vi "Write Output waveform.vi"(8 "error in (no error)":errorcluster, 10 "Output waveform":i16[](array[numeric]), 11 "RP I-V Driver in":refnum<class "RP I-V Driver.lvclass">) -> (0 "error out":errorcluster, 3 "RP I-V Driver out":refnum<class "RP I-V Driver.lvclass">)   [LabVIEW 2016, in "RP I-V Driver.lvclass"]
uses:
  RP I-V Driver.lvclass
  RP I-V Driver.lvclass/RP I-V Driver.ctl
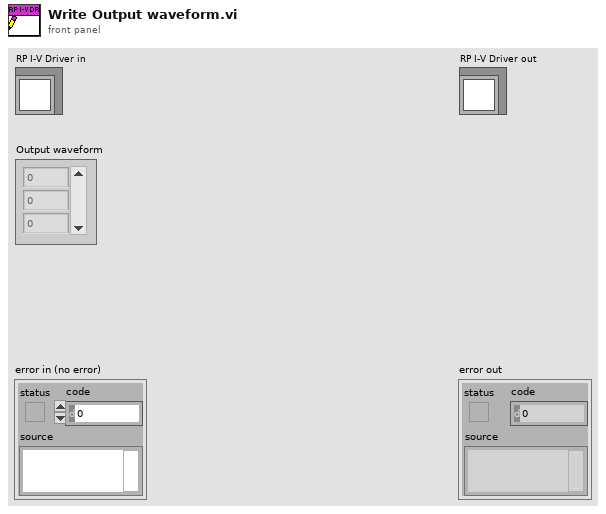
[diagram p1: front panel]
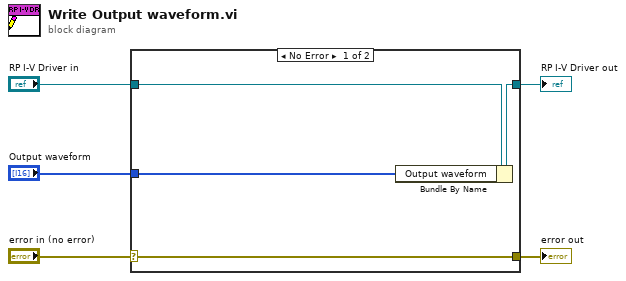
[diagram p0: block diagram]
diagram:
  n1 = case shown="No Error" "error in (no error)" {
    selector: "error in (no error)" -> [w9 w10]
    tunnel: [w9 w10] -> w4
    tunnel: [w7 w11] -> w2
    tunnel: "RP I-V Driver in" -> [w8 w11]
    tunnel: "Output waveform" -> [w6 _]
    frame No Error {
      n2 = Bundle By Name(cluster=w8, "Output waveform"=w6) -> (w7:refnum<class "RP I-V Driver.lvclass">)
    }
    frame Error {
    }
  }
  "error out" <- w4
  "RP I-V Driver out" <- w2
